vi "get index of tag read by channel.vi"(9 "channel":string, 10 "module guid":string, 11 "readers":T1[](array[typedef])) -> (3 "tag index":i32)   [LabVIEW 2014, in "engine configuration.lvclass"]
uses:
  engine configuration.lvclass
  module channel pairings.ctl
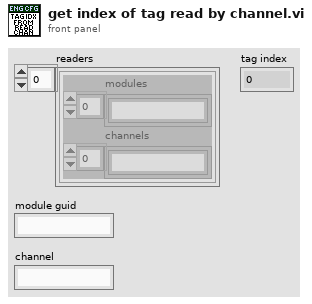
[diagram p1: front panel]
types:
  T1 = typedef "engine configuration.lvclass/module channel pairings.ctl" = cluster{"modules":string[], "channels":string[]}
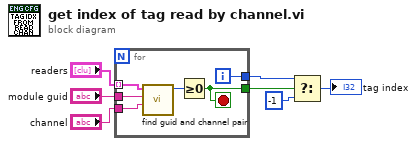
[diagram p0: block diagram]
diagram:
  n1 = for {
    tunnel: [w12] -> w4
    tunnel: "readers" -> [w11] mode=indexing
    tunnel: "module guid" -> [w10]
    tunnel: "channel" -> [w9]
    tunnel: [w8] -> w6
    i -> [w12]
    stop <- w8 stop-if-true
    n2 = call "find guid and channel pair.vi"("channel name"=w9, "Module GUID"=w10, "listing"=w11) -> ("index"=w13:i32)  [unwired: 8 in]
    n3 = Greater Or Equal To 0?(x=w13) -> (x >= 0?=w8:bool)
  }
  n4 = Select(t=w4, s=w6, f=-1) -> (s? t:f=→"tag index":i32)
